vi "Get Attention from USB port.vi"(8 "error in (no error)":errorcluster, 11 "VISA resource name":refnum<visa-resource-name>) -> (0 "error out":errorcluster, 3 "VISA resource name out":refnum<visa-resource-name>)   [LabVIEW 2016]
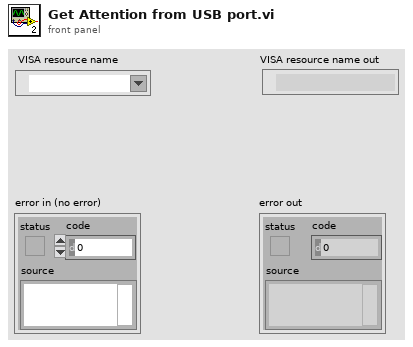
[diagram p1: front panel]
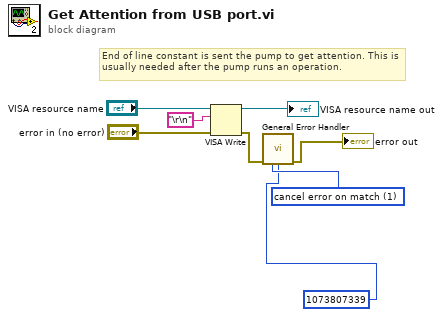
[diagram p0: block diagram]
diagram:
  w2 = 1 items=["no exception", "cancel error on match", "set error on match"] ("[exception action] (none:0)")
  # "End of line constant is sent the pump to get attention. This is usually needed after the pump runs an operation."
  n1 = VISA Write(VISA resource name="VISA resource name", write buffer="\r\n", error in (no error)="error in (no error)") -> (VISA resource name out=→"VISA resource name out":refnum<visa-resource-name>, error out=w4:errorcluster)  [unwired: 1 out]
  n2 = call <vilib>:"General Error Handler.vi"("error in (no error)"=w4, "[exception action] (none:0)"=w2, "[exception code]"=1073807339) -> ("error out"=→"error out":errorcluster)  [unwired: 8 in, 4 out]
